vi "GetEquipNames.vi"(11 "AssetNodes":T1[](array[typedef])) -> (3 "equip names":variant)   [LabVIEW 2016]
doc: "Gets equipment names from the asset nodes."
uses:
  <vilib>/addons/InsightCM/MessageBus/Base/controls/AssetState.ctl
  <vilib>/addons/InsightCM/MessageBus/Base/controls/KeyValuePair.ctl
  <vilib>/addons/InsightCM/MessageBus/Base/controls/Metric.ctl
  <vilib>/addons/InsightCM/MessageBus/Base/controls/AssetNodeReference.ctl
  <vilib>/addons/InsightCM/MessageBus/Base/controls/AssetNodeView.ctl
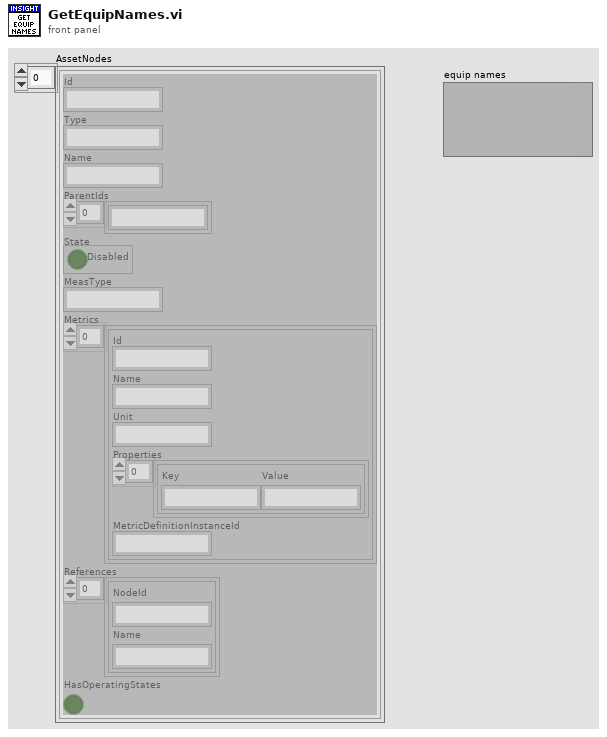
[diagram p1: front panel]
types:
  T1 = typedef "AssetNodeView.ctl" = cluster{"Id":string, "Type":string, "Name":string, "ParentIds":string[], "State":T2, "MeasType":string, "Metrics":T3[], "References":T5[], "HasOperatingStates":bool}
  T2 = typedef "AssetState.ctl" = cluster{"Disabled":bool}
  T3 = typedef "Metric.ctl" = cluster{"Id":string, "Name":string, "Unit":string, "Properties":T4[], "MetricDefinitionInstanceId":string}
  T4 = typedef "KeyValuePair.ctl" = cluster{"Key":string, "Value":string}
  T5 = typedef "AssetNodeReference.ctl" = cluster{"NodeId":string, "Name":string}
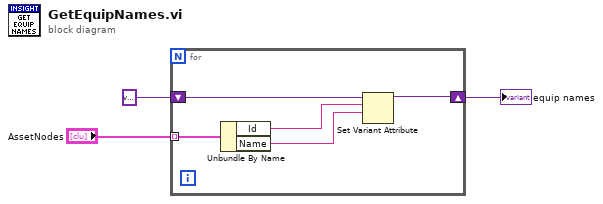
[diagram p0: block diagram]
diagram:
  n1 = for {
    tunnel: "AssetNodes" -> [w8] mode=indexing
    shift-right: [w7] -> w1
    shift-left: variant ("trend names") -> [w5]
    n2 = Unbundle By Name(w8) -> ("Id"=w6:string, "Name"=w4:string)
    n3 = Set Variant Attribute(Variant=w5, name=w6, value=w4) -> (Variant out=w7:variant)  [unwired: 1 in, 2 out]
  }
  "equip names" <- w1
